vi "Write WorkDir.vi"(8 "error in (no error)":errorcluster, 10 "Work Dir":path, 11 "HIJ Vision Camera App in":refnum<class "HIJ Vision Camera App.lvclass">) -> (0 "error out":errorcluster, 3 "HIJ Vision Camera App out":refnum<class "HIJ Vision Camera App.lvclass">)   [LabVIEW 2020, in "HIJ Vision Camera App.lvlib" / "HIJ Vision Camera App.lvclass"]
uses:
  HIJ Vision Camera App.lvclass
  HIJ Vision Application/HIJ Vision Application/HIJ Vision Application.lvclass
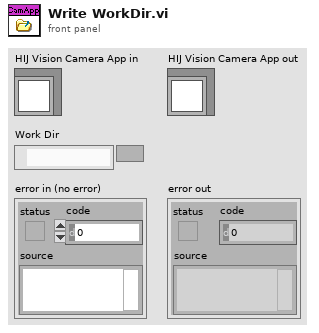
[diagram p1: front panel]
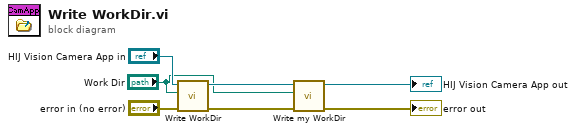
[diagram p0: block diagram]
diagram:
  n1 = call-parent "Write WorkDir.vi"("error in (no error)"="error in (no error)", "Work Dir"="Work Dir", "HIJ Vision Application in"="HIJ Vision Camera App in") -> ("error out"=w2:errorcluster, "HIJ Vision Application out"=w5:refnum<class "HIJ Vision Camera App.lvclass">)  [unwired: 7 in]
  n2 = call "Write my WorkDir.vi"("error in (no error)"=w2, "Work Dir"="Work Dir", "HIJ Vision Camera App in"=w5) -> ("error out"=→"error out":errorcluster, "HIJ Vision Camera App out"=→"HIJ Vision Camera App out":refnum<class "HIJ Vision Camera App.lvclass">)  [unwired: 7 in]
